vi "U Boat form command string.vi"(0 "Jib Sheet":u16=1500, 1 "Rudder":u16=1500, 2 "Main sheet":u16=1500) -> (4 "Jib":u16, 5 "Rudder":u16, 6 "String":string="$CR1500M1500J1500\n", 7 "Main":u16)   [LabVIEW 2013]
doc: "This VI takes in servo values for Rudder, Main Sheet, and Jib Sheet and creates a command string to be sent to the Arbotix-M PCB via the XBee link."
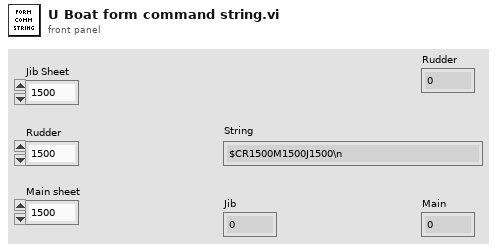
[diagram p1: front panel]
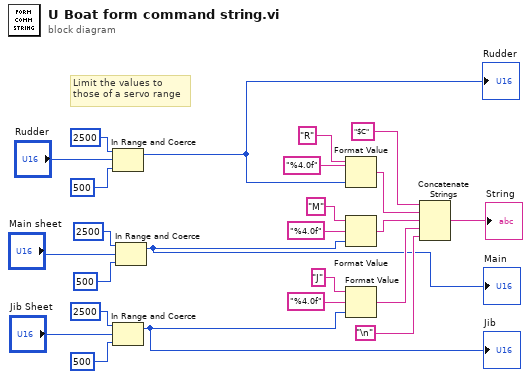
[diagram p0: block diagram]
diagram:
  # "Limit the values to \nthose of a servo range"
  n1 = In Range and Coerce(upper limit=u16 2500, x="Rudder", lower limit=u16 500) -> (coerced(x)=w5:u16)  [unwired: 1 out]
  "Rudder" <- w5
  n2 = In Range and Coerce(upper limit=u16 2500, x="Jib Sheet", lower limit=u16 500) -> (coerced(x)=w1:u16)  [unwired: 1 out]
  "Jib" <- w1
  n3 = In Range and Coerce(upper limit=u16 2500, x="Main sheet", lower limit=u16 500) -> (coerced(x)=w3:u16)  [unwired: 1 out]
  "Main" <- w3
  n4 = Format Value(string ("")="R", format string="%4.0f", value (0)=w5) -> (output string=w21:string)
  n5 = Format Value(string ("")="M", format string="%4.0f", value (0)=w3) -> (output string=w16:string)
  n6 = Format Value(string ("")="J", format string="%4.0f", value (0)=w1) -> (output string=w15:string)
  n7 = Concatenate Strings("$C", w21, w16, w15, "\n") -> (→"String":string)
